vi "setValveArduinoNew.vi"(8 "value":u8, 11 "valve id":i32) -> ()   [LabVIEW 2012]
uses:
  GlobalArduinoNew.vi
  <vilib>/LabVIEW Interface for Arduino/LabVIEW Interface for Arduino.lvlib
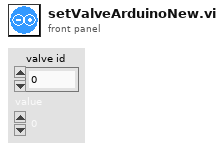
[diagram p1: front panel]
types:
  T1 = typedef "Semaphore RefNum" = refnum<k1>
  T2 = typedef "LabVIEW Interface for Arduino.lvlib/Arduino Resource.ctl" = cluster{"VISA resource":refnum<visa-resource-name>, "Board Type":T3, "Connection Type":enum8{"USB / Serial"}, "Bytes Per Packet (15)":u8}
  T3 = typedef "LabVIEW Interface for Arduino.lvlib/Board Type.ctl" = enum16{"Uno", "Dimuelanove w/Atmega 328", "Mega 2560"}
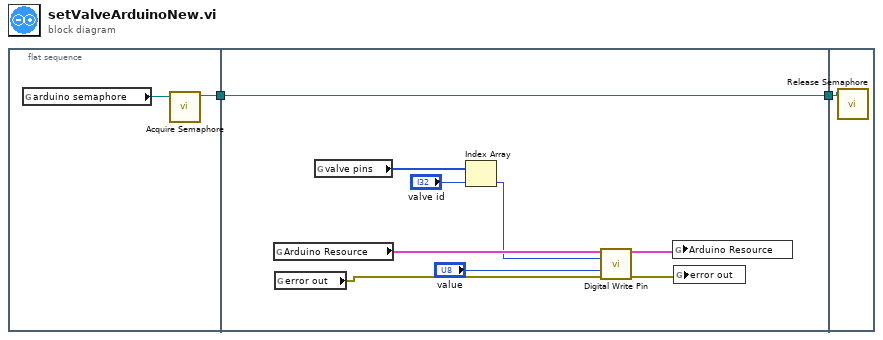
[diagram p0: block diagram]
diagram:
  n1 = flat-sequence {
    tunnel: [w3] -> w1
    tunnel: [w5] -> w2
    tunnel: w1 -> [w5]
    tunnel: w2 -> [w14]
    frame #0 {
      n2 = global read "GlobalArduinoNew.vi" "arduino semaphore"() -> (w4:T1)
      n3 = call <vilib>:"Acquire Semaphore.vi"("semaphore"=w4) -> ("semaphore out"=w3:T1)  [unwired: 4 in, 2 out]
    }
    frame #1 {
      n4 = global read "GlobalArduinoNew.vi" "Arduino Resource"() -> (w13:T2)
      n5 = global read "GlobalArduinoNew.vi" "error out"() -> (w12:errorcluster)
      n6 = global read "GlobalArduinoNew.vi" "valve pins"() -> (w11:u8[])
      n7 = Index Array(array=w11, index="valve id") -> (element=w9:u8)
      n8 = call <vilib>:"Digital Write Pin.vi"("Arduino Resource"=w13, "Digital I/O Pin (0)"=w9, "Value (0)"="value", "error in"=w12) -> ("Arduino Resource"=w7:T2, "error out"=w6:errorcluster)  [unwired: 10 in]
      n9 = global write "GlobalArduinoNew.vi" "Arduino Resource"(w7) -> ()
      n10 = global write "GlobalArduinoNew.vi" "error out"(w6) -> ()
    }
    frame #2 {
      n11 = call <vilib>:"Release Semaphore.vi"("semaphore"=w14) -> ()  [unwired: 5 in, 2 out]
    }
  }
